vi "getBroadcastData-system.vi"(8 "error in (no error)":errorcluster, 10 "Device index":i32, 11 "SM1000-control in":T2) -> (0 "error out":errorcluster, 2 "System information":T1, 3 "SM1000-control out":T2)   [LabVIEW 2013, in "MaterialCharacterization.lvlib" / "MC-SM1000.lvclass"]
doc: "Get embedded controller device data.\n\nThis function is used by a client application to retrieve various types of data related to the specified EC1000 module. This particular function retreives the 'System' data."
uses:
  MC-SM1000.lvclass
  Object-reference.ctl
  System-information.ctl
  MC-SM1000.lvclass/MC-SM1000.ctl
  Custom-errors.ctl
  Device-data-types.ctl
  C:/Users/vangeste/Desktop/2015-06-02 - SLM - MAIF/HC-HardwareCharacterization/Sources/SM1000/LECBroadcast.dll
  HC-HardwareCharacterization/Sources/SM1000/LECBroadcast.dll
  DOTNET-error-int.vi
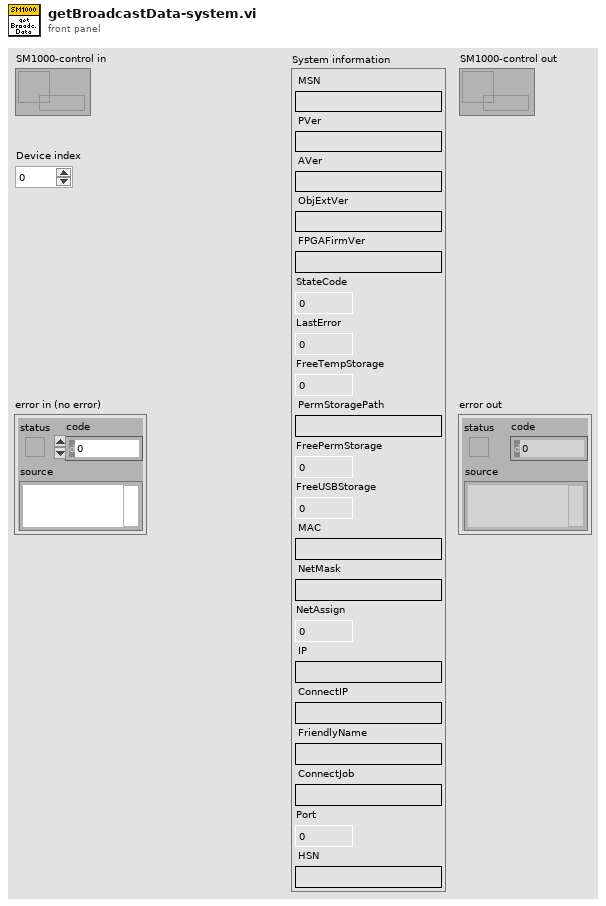
[diagram p1: front panel]
types:
  T1 = typedef "MaterialCharacterization.lvlib/MC-SM1000.lvclass/System-information.ctl" = cluster{"MSN":string, "PVer":string, "AVer":string, "ObjExtVer":string, "FPGAFirmVer":string, "StateCode":u32, "LastError":i32, "FreeTempStorage":u32, "PermStoragePath":string, "FreePermStorage":u32, "FreeUSBStorage":u32, "MAC":string, "NetMask":string, "NetAssign":i32, "IP":string, "ConnectIP":string, "FriendlyName":string, "ConnectJob":string, "Port":u32, "HSN":string}
  T2 = typedef "MaterialCharacterization.lvlib/MC-SM1000.lvclass/Object-reference.ctl" = refnum<data-value>
  T3 = typedef "MaterialCharacterization.lvlib/MC-SM1000.lvclass/Custom-errors.ctl" = enum16{"No error", "Not implemented", "Command not recognized", "Invalid input", "No connection", "Timeout", "Resource not loaded"}
  T4 = typedef "MaterialCharacterization.lvlib/MC-SM1000.lvclass/Device-data-types.ctl" = i32
  T5 = typedef "MaterialCharacterization.lvlib/MC-SM1000.lvclass/Device-identification.ctl" = cluster{"Name":string, "IP":string, "Mac address":string}
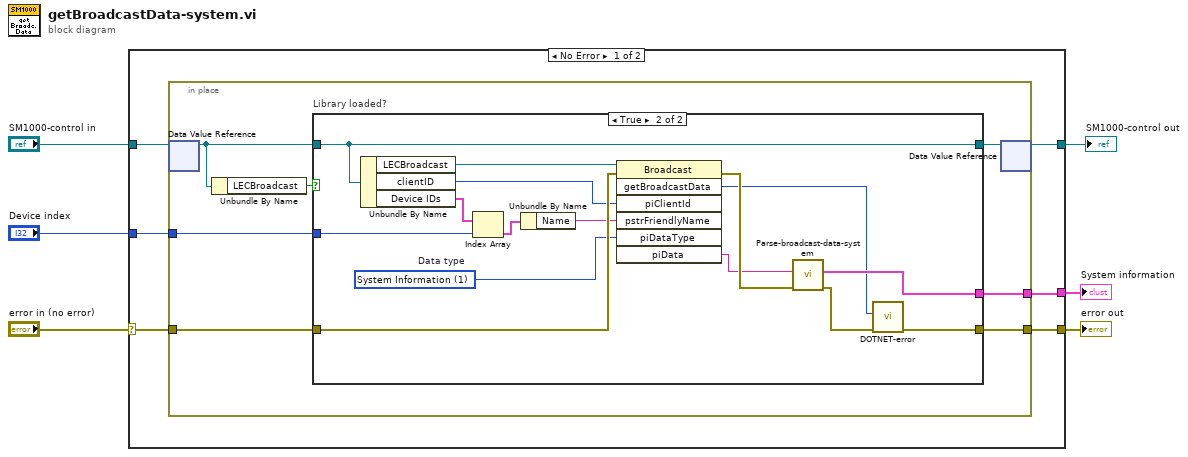
[diagram p0: block diagram]
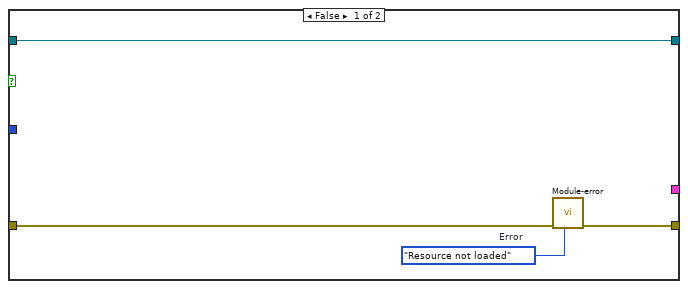
[diagram p2: hidden frame]
diagram:
  n1 = case shown="No Error" "error in (no error)" {
    selector: "error in (no error)" -> [w10 w40]
    tunnel: [w9 w40] -> w5
    tunnel: [w11 w39] -> w3
    tunnel: "SM1000-control in" -> [w12 w39]
    tunnel: [w8 _] -> w2
    tunnel: "Device index" -> [w7 _]
    frame No Error {
      n2 = in-place {
        in-place-border: w10 -> [w19]
        in-place-border: [w16] -> w9
        in-place-border: [w14] -> w8
        in-place-border: w7 -> [w13]
        n3 = in-place-dvr #1(w12) -> (w17:refnum<class "MC-SM1000.lvclass">)  [unwired: 1 out]
        n4 = Unbundle By Name(w17) -> ("LECBroadcast"=w18:bool)
        n5 = case "Library loaded?" shown="True" w18 {
          tunnel: w19 -> [w23 w37]
          tunnel: w17 -> [w21 w29]
          tunnel: [w22 w26] -> w16
          tunnel: [w21 w29] -> w15
          tunnel: [_ w28] -> w14
          tunnel: w13 -> [_ w33]
          frame False {
            w20 = Custom-errors."Resource not loaded"  # Error
            n6 = call "Module-error.vi"("Error"=w20, "error in (no error)"=w23) -> ("error out"=w22:errorcluster)  [unwired: 9 in]
          }
          frame True {
            w27 = T4 1 items=["System Information"=1, "Status Information"=7]  # Data type
            n7 = Unbundle By Name(w29) -> ("LECBroadcast"=w38:refnum<k24>, "clientID"=w36:i32, "Device IDs"=w34:T5[])
            n8 = Index Array(array=w34, index=w33) -> (element=w31:T5)
            n9 = Unbundle By Name(w31) -> ("Name"=w32:string)
            n10 = invoke class="Broadcast" method="getBroadcastData"(reference=w38, error in=w37, "piClientId"=w36, "pstrFriendlyName"=w32, "piDataType"=w27) -> (error out=w35:errorcluster, "getBroadcastData"=w24:u32, "piData"=w30:string)  [unwired: 2 in, 4 out]
            n11 = call "Parse-broadcast-data-system.vi"("error in (no error)"=w35, "Multiple device identification XML string"=w30) -> ("error out"=w25:errorcluster, "System information"=w28:T1)  [unwired: 8 in]
            n12 = call-poly "DOTNET-error.vi"("error in (no error)"=w25, "Retun code"=w24) -> ("error out"=w26:errorcluster)  [unwired: 9 in]
          }
        }
        n13 = in-place-dvr #1(w15) -> (w11:T2)  [unwired: 1 out]
      }
    }
    frame Error {
    }
  }
  "error out" <- w5
  "SM1000-control out" <- w3
  "System information" <- w2
